vi "Write Config.vi"(8 "error in (no error)":errorcluster, 10 "Config":variant, 11 "HtmlReportPlugin in":refnum<class "HtmlReportPlugin.lvclass">) -> (0 "error out":errorcluster, 3 "HtmlReportPlugin out":refnum<class "HtmlReportPlugin.lvclass">)   [LabVIEW 2015, in "HtmlReportPlugin.lvclass"]
uses:
  HtmlReportPlugin.lvclass
  HtmlReportPlugin.lvclass/HtmlReportPlugin.ctl
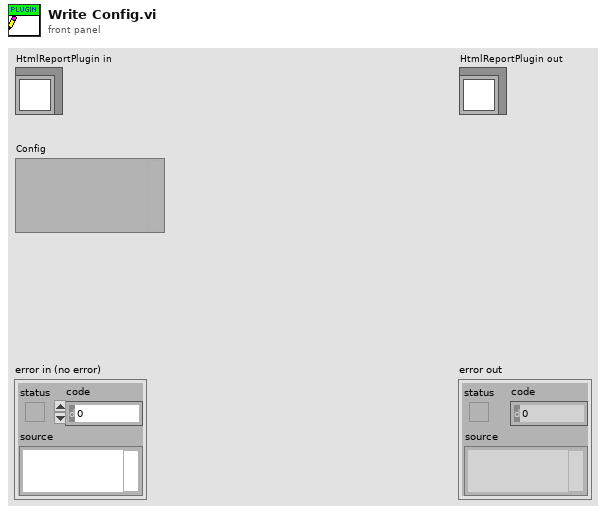
[diagram p1: front panel]
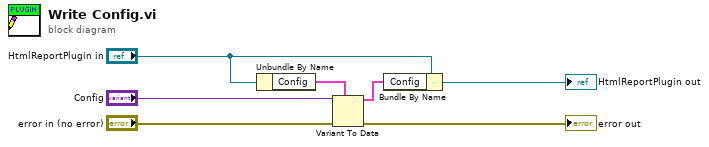
[diagram p0: block diagram]
diagram:
  n1 = Unbundle By Name("HtmlReportPlugin in") -> ("Config"=w7:cluster{"Enable":bool, "Report Folder":string})
  n2 = Variant To Data(error in="error in (no error)", type=w7, Variant="Config") -> (data=w6:cluster{"Enable":bool, "Report Folder":string}, error out=→"error out":errorcluster)
  n3 = Bundle By Name(cluster="HtmlReportPlugin in", "Config"=w6) -> (→"HtmlReportPlugin out":refnum<class "HtmlReportPlugin.lvclass">)
